vi "LEDs Vi.vi"(4 "LED Control Type":T1) -> (0 "G":dbl, 1 "B":dbl, 2 "R":dbl)   [LabVIEW 2017]
uses:
  LED Control Type.ctl
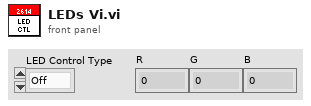
[diagram p1: front panel]
types:
  T1 = typedef "LED Control Type.ctl" = enum16{"Off", "Waiting On Field", "Connected ", "Cube In Intake", "Climbing", "Auto Cube Capture", "Ready for Cube Floor", "Ready for Cube Portal"}
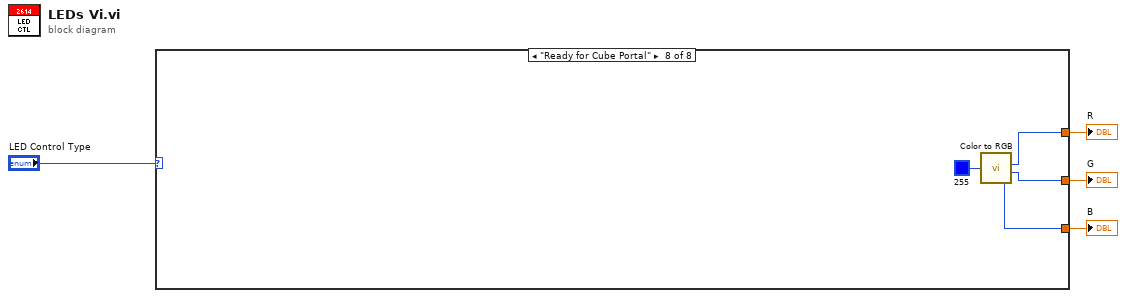
[diagram p0: block diagram]
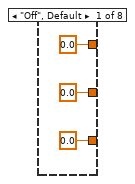
[diagram p2: hidden frame]
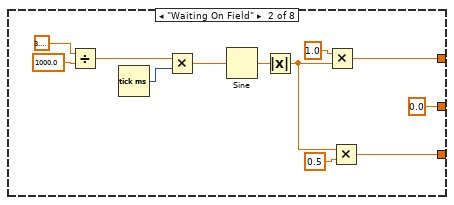
[diagram p3: hidden frame]
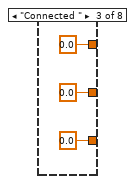
[diagram p4: hidden frame]
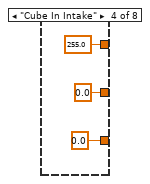
[diagram p5: hidden frame]
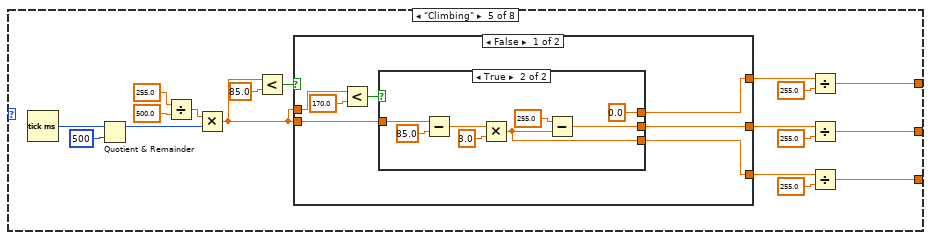
[diagram p6: hidden frame]
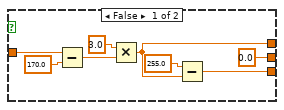
[diagram p7: hidden frame]
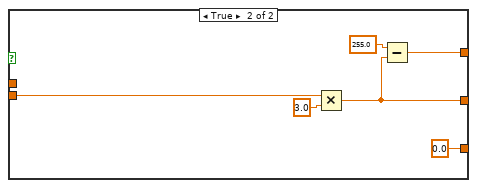
[diagram p8: hidden frame]
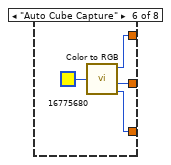
[diagram p9: hidden frame]
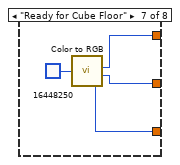
[diagram p10: hidden frame]
diagram:
  n1 = case shown="\"Ready for Cube Portal\"" "LED Control Type" {
    tunnel: [0.0 ("Percent Output") w9 0.0 ("Percent Output") 255.0 ("Percent Output") w33 w75 w79 w83] -> w4
    tunnel: [0.0 ("Percent Output") w11 0.0 ("Percent Output") 0.0 ("Percent Output") w32 w73 w77 w81] -> w2
    tunnel: [0.0 ("Percent Output") 0.0 ("Percent Output") 0.0 ("Percent Output") 0.0 ("Percent Output") w29 w74 w78 w82] -> w3
    frame "Off", Default {
    }
    frame "Waiting On Field" {
      n2 = Divide(x=3.141592653589793, y=1000.0) -> (x/y=w18:dbl)
      n3 = Tick Count (ms)() -> (millisecond timer value=w17:u32)
      n4 = Multiply(x=w18, y=w17) -> (x*y=w19:dbl)
      n5 = Sine(x=w19) -> (sin(x)=w15:dbl)
      n6 = Absolute Value(x=w15) -> (abs(x)=w16:dbl)
      n7 = Multiply(x=1.0, y=w16) -> (x*y=w9:dbl)
      n8 = Multiply(x=w16, y=0.5) -> (x*y=w11:dbl)
    }
    frame "Connected " {
    }
    frame "Cube In Intake" {
    }
    frame "Climbing" {
      n9 = Tick Count (ms)() -> (millisecond timer value=w43:u32)
      n10 = Quotient & Remainder(x=w43, y=u32 500) -> (x-y*floor(x/y)=w41:u32)  [unwired: 1 out]
      n11 = Divide(x=255.0, y=500.0) -> (x/y=w40:dbl)
      n12 = Multiply(x=w40, y=w41) -> (x*y=w35:dbl)
      n13 = Less?(x=w35, y=85.0) -> (x < y?=w36:bool)
      n14 = case shown="False" w36 {
        tunnel: w35 -> [w47 w72]
        tunnel: [w46 w69] -> w34
        tunnel: [w45 0.0] -> w31
        tunnel: [w44 w67] -> w30
        tunnel: w35 -> [w49 _]
        frame False {
          n15 = Less?(x=w49, y=170.0) -> (x < y?=w50:bool)
          n16 = case shown="True" w50 {
            tunnel: w47 -> [w58 w66]
            tunnel: [w53 0.0] -> w46
            tunnel: [w52 w60] -> w45
            tunnel: [0.0 w59] -> w44
            frame False {
              n17 = Subtract(x=w58, y=170.0) -> (x-y=w55:dbl)
              n18 = Multiply(x=3.0, y=w55) -> (x*y=w53:dbl)
              n19 = Subtract(x=255.0, y=w53) -> (x-y=w52:dbl)
            }
            frame True {
              n20 = Subtract(x=w66, y=85.0) -> (x-y=w62:dbl)
              n21 = Multiply(x=w62, y=3.0) -> (x*y=w60:dbl)
              n22 = Subtract(x=255.0, y=w60) -> (x-y=w59:dbl)
            }
          }
        }
        frame True {
          n23 = Multiply(x=w72, y=3.0) -> (x*y=w67:dbl)
          n24 = Subtract(x=255.0, y=w67) -> (x-y=w69:dbl)
        }
      }
      n25 = Divide(x=w34, y=255.0) -> (x/y=w33:dbl)
      n26 = Divide(x=w30, y=255.0) -> (x/y=w29:dbl)
      n27 = Divide(x=w31, y=255.0) -> (x/y=w32:dbl)
    }
    frame "Auto Cube Capture" {
      n28 = call <vilib>:"Color to RGB.vi"("Color"=u32 16775680) -> ("Resolved Color"=w75:u32, "G"=w74:u8, "B"=w73:u8)  [unwired: 1 out]
    }
    frame "Ready for Cube Floor" {
      n29 = call <vilib>:"Color to RGB.vi"("Color"=u32 16448250) -> ("R"=w79:u8, "G"=w78:u8, "B"=w77:u8)  [unwired: 1 out]
    }
    frame "Ready for Cube Portal" {
      n30 = call <vilib>:"Color to RGB.vi"("Color"=u32 255) -> ("R"=w83:u8, "G"=w82:u8, "B"=w81:u8)  [unwired: 1 out]
    }
  }
  "R" <- w4
  "G" <- w3
  "B" <- w2
